vi "Get Single-Multiple Statistics Measurement.vi"(6 "Measurement Group Size":enum16{"Single", "Multiple"}(ring), 8 "error in (no error)":errorcluster, 11 "MSOX6004 in":refnum<class "MSOX6004.lvclass">) -> (0 "error out":errorcluster, 2 "Statistics":T1(array[cluster]), 3 "MSOX6004 out":refnum<class "MSOX6004.lvclass">)   [LabVIEW 2018, in "MSOX6004.lvlib" / "MSOX6004.lvclass"]
uses:
  MSOX6004.lvclass
  <instrlib>/Keysight InfiniiVision/Keysight InfiniiVision.lvlib
  PPLs/Oscilloscope/Parent/Oscilloscope.lvlibp/Oscilloscope.lvclass
  C:/Projects/LabVIEW/PPLs/Oscilloscope/Parent/Oscilloscope.lvlibp/Oscilloscope.lvclass
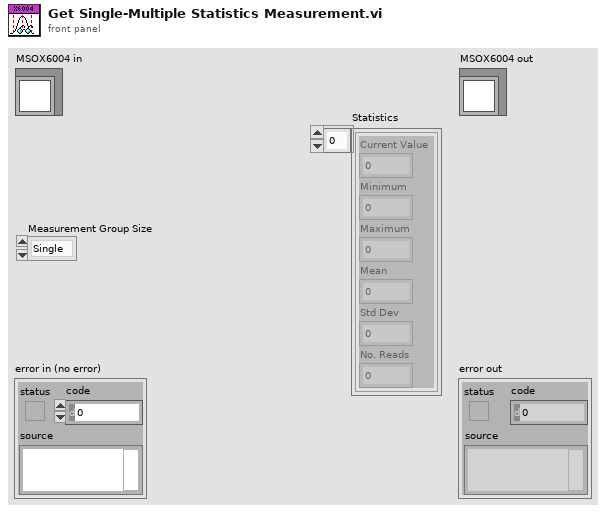
[diagram p1: front panel]
types:
  T1 = cluster{"Current Value":dbl, "Minimum":dbl, "Maximum":dbl, "Mean":dbl, "Std Dev":dbl, "No. Reads":dbl}[]
  T2 = cluster{"Current Value":dbl, "Minimum":dbl, "Maximum":dbl, "Mean":dbl, "Std Dev":dbl, "No. Reads":dbl}
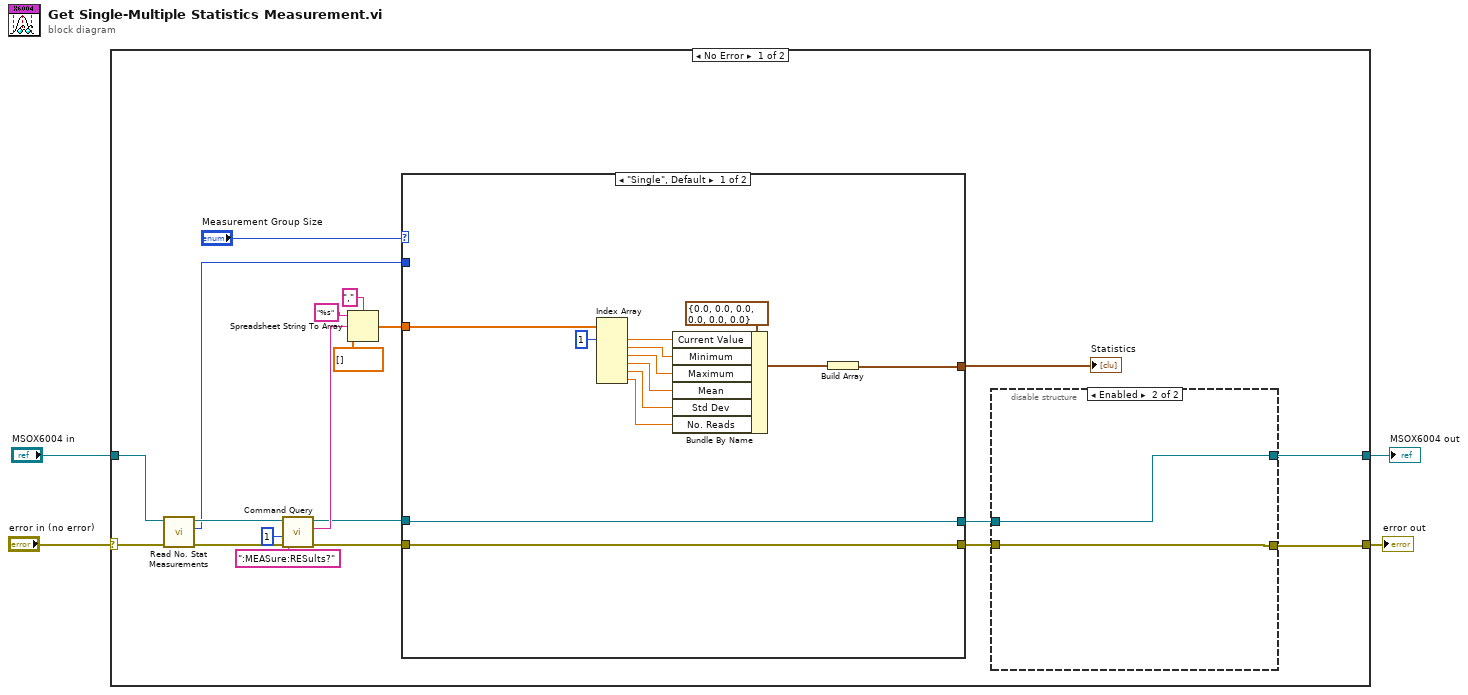
[diagram p0: block diagram]
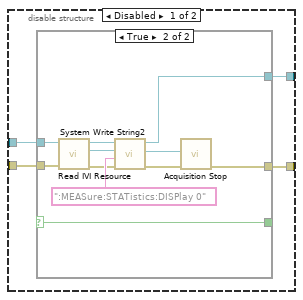
[diagram p2: hidden frame]
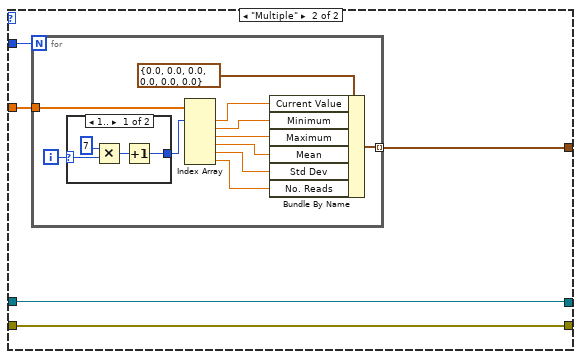
[diagram p4: hidden frame]
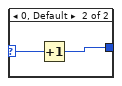
[diagram p5: hidden frame]
diagram:
  n1 = case shown="No Error" "error in (no error)" {
    selector: "error in (no error)" -> [w20 w79]
    tunnel: "MSOX6004 in" -> [w21 w80]
    tunnel: [w23 w80] -> w2
    tunnel: [w22 w79] -> w1
    frame No Error {
      n2 = call "Read No. Stat Measurements.vi"("error in (no error)"=w20, "Oscilloscope in"=w21) -> ("error out"=w18:errorcluster, "No. Stat Measurements"=w10:u32, "Oscilloscope out"=w19:refnum<class "MSOX6004.lvclass">)  [unwired: 7 in]
      n3 = call "Command Query.vi"("error in (no error)"=w18, "Delay (ms)"=u32 1, "Command"=":MEASure:RESults?", "MSOX6004 in"=w19) -> ("error out"=w24:errorcluster, "Response"=w11:string, "MSOX6004 out"=w5:refnum<class "MSOX6004.lvclass">)  [unwired: 5 in]
      n4 = Spreadsheet String To Array(delimiter (Tab)=",", format string="%s", spreadsheet string=w11, array type (2D Dbl)=dbl[] []) -> (array=w16:dbl[])
      n5 = case shown="\"Single\", Default" "Measurement Group Size" {
        tunnel: w24 -> [w45 w58]
        tunnel: w16 -> [w48 w61]
        tunnel: w10 -> [_ w60]
        tunnel: [w46 w59] -> w8
        tunnel: [w45 w58] -> w7
        tunnel: [w44 w57] -> w6
        tunnel: w5 -> [w44 w57]
        frame "Single", Default {
          n6 = Index Array(array=w48, index #1=1 ("index")) -> (element #1=w54:dbl, element #2=w53:dbl, element #3=w52:dbl, element #4=w51:dbl, element #5=w50:dbl, element #6=w49:dbl)  [unwired: 5 in]
          n7 = Bundle By Name(cluster=T2 {"Current Value"=0.0, "Minimum"=0.0, "Maximum"=0.0, "Mean"=0.0, "Std Dev"=0.0, "No. Reads"=0.0} ("Statistics"), "Current Value"=w54, "Minimum"=w53, "Maximum"=w52, "Mean"=w51, "Std Dev"=w50, "No. Reads"=w49) -> (w47:T2)
          n8 = Build Array(w47) -> (w46:T1)
        }
        frame "Multiple" {
          n9 = for {
            N: w60 -> [_]
            tunnel: w61 -> [w72]
            tunnel: [w62] -> w59 mode=indexing
            i -> [w71]
            n10 = case shown="1.." w71 {
              selector: w71 -> [w76 w78]
              tunnel: [w73 w77] -> w70
              frame 1.. {
                n11 = Multiply(x=7, y=w76) -> (x*y=w74:i32)
                n12 = Increment(x=w74) -> (x+1=w73:i32)
              }
              frame 0, Default {
                n13 = Increment(x=w78) -> (x+1=w77:i32)
              }
            }
            n14 = Index Array(array=w72, index #1=w70) -> (element #1=w68:dbl, element #2=w67:dbl, element #3=w66:dbl, element #4=w65:dbl, element #5=w64:dbl, element #6=w63:dbl)  [unwired: 5 in]
            n15 = Bundle By Name(cluster=T2 {"Current Value"=0.0, "Minimum"=0.0, "Maximum"=0.0, "Mean"=0.0, "Std Dev"=0.0, "No. Reads"=0.0} ("Statistics"), "Current Value"=w68, "Minimum"=w67, "Maximum"=w66, "Mean"=w65, "Std Dev"=w64, "No. Reads"=w63) -> (w62:T2)
          }
        }
      }
      "Statistics" <- w8
      n16 = disable-structure shown="Enabled" {
        disable-tunnel: [w28 w42] -> w23
        disable-tunnel: [w27 w43] -> w22
        disable-tunnel: w7 -> [w26 w43]
        disable-tunnel: w6 -> [w25 w42]
        frame Disabled {
          n17 = case shown="True" {
            selector: _ -> [w29 w32]
            tunnel: [w31 w36] -> w28
            tunnel: [w30 w35] -> w27
            tunnel: w26 -> [w30 w34]
            tunnel: w25 -> [w31 w33]
            tunnel: [w29 w32] -> _
            frame False {
            }
            frame True {
              n18 = call "Read IVI Resource.vi"("error in (no error)"=w34, "MSOX6004 in"=w33) -> ("error out"=w38:errorcluster, "IVI Resource"=w41:refnum<k15>, "MSOX6004 out"=w36:refnum<class "MSOX6004.lvclass">)  [unwired: 7 in]
              n19 = call <instrlib>:"System Write String2.vi"("error in (no error)"=w38, "Data"=":MEASure:STATistics:DISPlay 0", "instrument handle"=w41) -> ("error out"=w37:errorcluster, "instrument handle out"=w39:refnum<k15>)  [unwired: 7 in]
              n20 = call <instrlib>:"Acquisition Stop.vi"("error in (no error)"=w37, "instrument handle"=w39) -> ("error out"=w35:errorcluster)  [unwired: 8 in, 1 out]
            }
          }
        }
        frame Enabled {
        }
      }
    }
    frame Error {
    }
  }
  "error out" <- w1
  "MSOX6004 out" <- w2
